vi "Get Device Adress.vi"(4 "error in (no error)":errorcluster, 7 "VISA resource name":refnum<visa-resource-name>) -> (0 "error out":errorcluster, 2 "Adress Number":i32, 3 "VISA resource name out":refnum<visa-resource-name>)   [LabVIEW 2012, in "Newport ESP301.lvlib"]
doc: "Reads the device adress fur use with IEEE-488 or USB communication."
uses:
  Newport ESP301.lvlib
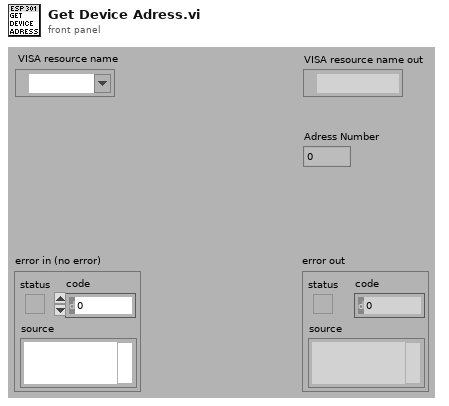
[diagram p1: front panel]
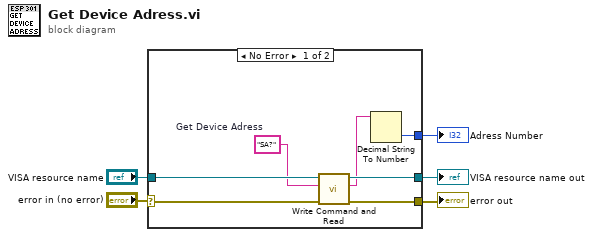
[diagram p0: block diagram]
diagram:
  n1 = case shown="No Error" "error in (no error)" {
    selector: "error in (no error)" -> [w9 w14]
    tunnel: [w11 w14] -> w5
    tunnel: "VISA resource name" -> [w12 w13]
    tunnel: [w10 w13] -> w4
    tunnel: [w7 _] -> w1
    frame No Error {
      w6 = "SA?"  # Get Device Adress
      n2 = call "Write Command and Read.vi"("error in (no error)"=w9, "Command"=w6, "VISA resource name"=w12) -> ("error out"=w11:errorcluster, "Returned string"=w8:string, "VISA resource name out"=w10:refnum<visa-resource-name>)  [unwired: 2 in, 2 out]
      n3 = Decimal String To Number(string=w8) -> (number=w7:i32)  [unwired: 2 in, 1 out]
    }
    frame Error {
    }
  }
  "error out" <- w5
  "VISA resource name out" <- w4
  "Adress Number" <- w1
